vi "Model OPCUA Check Status.vi"(8 "error in (no error)":errorcluster, 11 "Model in":refnum<class "Model.lvclass">) -> (0 "error out":errorcluster)   [LabVIEW 2021, in "Model.lvlib" / "Model.lvclass"]
uses:
  Model.lvclass
  Model.lvclass/Model.ctl
  c082fed2-e689-4666-b91a-ad6a0abfd1cc.vi
  cbdd33bf-e0af-482d-9349-bbda270fe613.vi
  <userlib>/John_Lib/AMC_FW/Read Next Message.vi
  <userlib>/John_Lib/AMC_FW/Parse State Queue__JKI.vi
  <userlib>/John_Lib/AMC_FW/Send Local Message.vi
  <userlib>/John_Lib/AMC_FW/Read Termination Message.vi
  <userlib>/John_Lib/AMC_FW/Create Single Message.vi
  <userlib>/John_Lib/AMC_FW/Update Message Routing Info.vi
  <userlib>/John_Lib/AMC_FW/Globals.vi
  <vilib>/Utility/error.llb/Trim Whitespace.vi
  <userlib>/John_Lib/AMC_FW/String to Array.vi
  <userlib>/John_Lib/AMC_FW/Send Message.vi
  <userlib>/John_Lib/AMC_FW/AMC_FW.lvlib
  <userlib>/John_Lib/OPCUA/OPCUA.lvclass
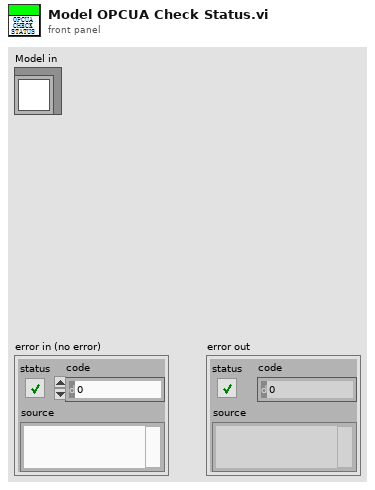
[diagram p1: front panel]
types:
  T1 = typedef "AMC_FW.lvlib/Queue.ctl" = cluster{"Q":T2, "Name":string}
  T2 = typedef "AMC_FW.lvlib/Message Queue.ctl" = refnum<queue>
  T3 = typedef "Model.lvlib/Model.lvclass/DVR.ctl" = cluster{"JKI_Network_Streams":refnum<class "NetworkConnection.lvclass">, "AMC Q":T4}
  T4 = typedef "Model.lvlib/Model.lvclass/AMC Q.ctl" = cluster{"Main":T1, "OPCUA":T1, "NetworkSteam":T1}
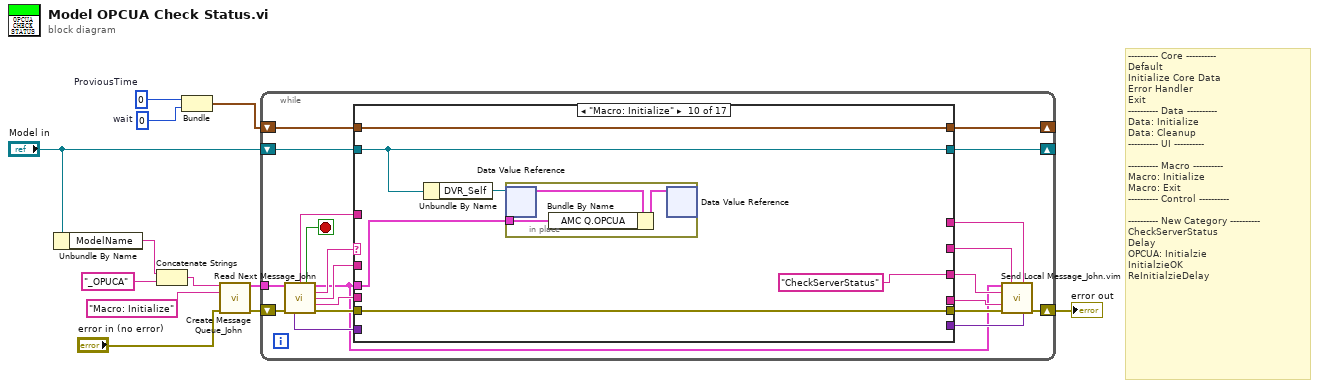
[diagram p0: block diagram]
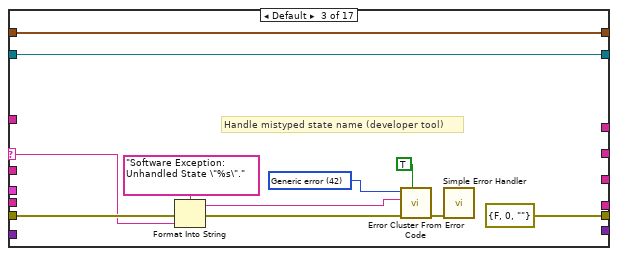
[diagram p4: hidden frame]
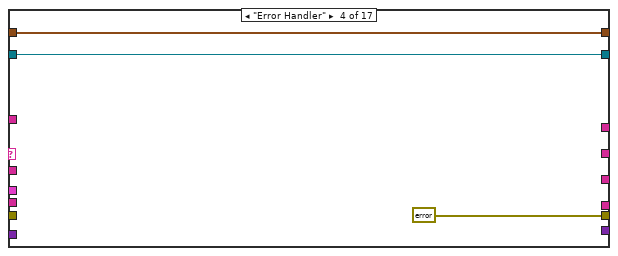
[diagram p5: hidden frame]
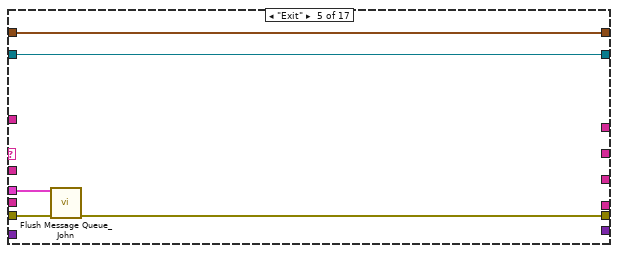
[diagram p6: hidden frame]
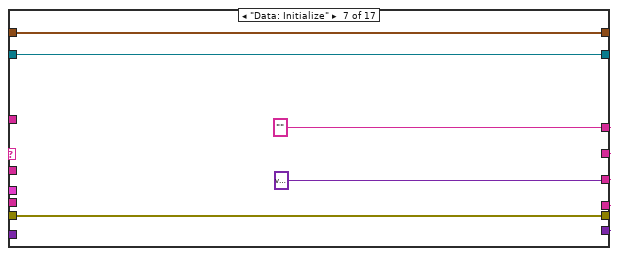
[diagram p8: hidden frame]
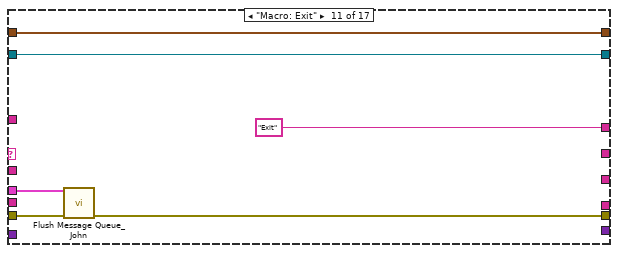
[diagram p11: hidden frame]
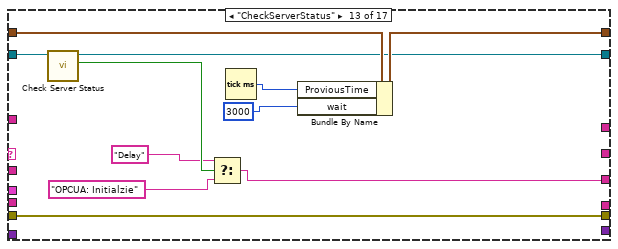
[diagram p13: hidden frame]
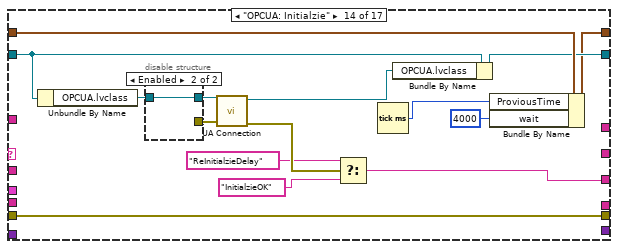
[diagram p14: hidden frame]
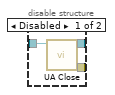
[diagram p15: hidden frame]
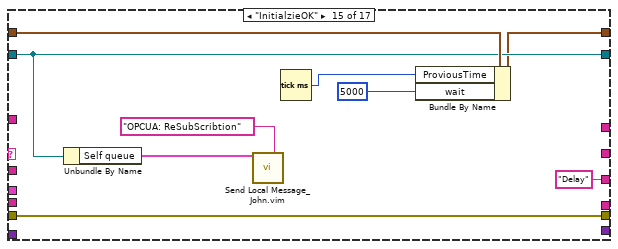
[diagram p16: hidden frame]
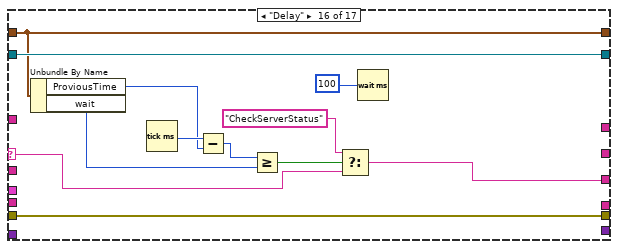
[diagram p17: hidden frame]
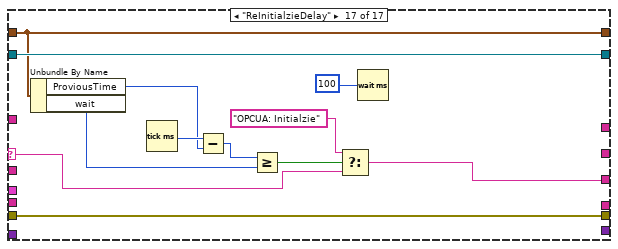
[diagram p18: hidden frame]
diagram:
  w1 = u32 0  # wait
  w11 = u32 0  # ProviousTime
  # "---------- Core ----------\nDefault\nInitialize Core Data\nError Handler\nExit\n---------- Data ----------\nData: Initialize\nData: Cleanup\n---------- UI ----------\n\n---------- Macro ----------\nMacro: Initialize\nMacro: Exit\n---------- Control ----------\n\n---------- New Category ----------\nCheckServerStatus\nDelay\nOPCUA: Initialzie\nInitialzieOK\nReInitialzieDelay"
  n1 = Unbundle By Name("Model in") -> ("ModelName"=w3:string)
  n2 = Concatenate Strings(w3, "_OPUCA" ("string")) -> (w9:string)
  n3 = Bundle("ProviousTime"=w11, "wait"=w1) -> (w10:cluster{"ProviousTime":u32, "wait":u32})  [unwired: 1 in]
  n4 = call <userlib>:"Create Message Queue_John.vi"("message queue name"=w9, "initial message names"="Macro: Initialize", "error in"="error in (no error)") -> ("message queue out"=w7:T1, "error out"=w6:errorcluster)  [unwired: 11 in]
  n5 = while {
    shift-right: [w24] -> w12
    shift-left: w6 -> [w32]
    shift-right: [w33] -> _
    shift-left: "Model in" -> [w26]
    tunnel: w7 -> [w29]
    shift-right: [w14] -> _
    shift-left: w10 -> [w15]
    stop <- w16 stop-if-true
    n6 = call <userlib>:"Read Next Message_John.vi"("Queue In"=w29, "error in"=w32) -> ("Previous State + Arguments"=w25:string, "exit process?"=w16:bool, "Queue Out"=w13:T1, "Current State"=w30:string, "Arguments"=w28:string, "message value"=w27:string, "variant"=w17:variant, "error out"=w31:errorcluster)  [unwired: 4 in, 2 out]
    n7 = case shown="\"Macro: Initialize\"" w30 {
      selector: w30 -> [_ _ w45 _ _ _ _ _ _ _ _ _ _ _ _ w133 w145]
      tunnel: w13 -> [_ _ _ _ w56 _ _ _ _ w73 w87 _ _ _ _ _ _]
      tunnel: w27 -> [_ _ _ _ _ _ _ _ _ _ _ _ _ _ _ _ _]
      tunnel: [w35 w39 errorcluster {"status"=FALSE, "code"=0, "source"=""} ("error out") errorcluster {"status"=FALSE, "code"=0, "source"=""} ("error out") w57 w60 w66 w68 w71 w78 w85 w90 w96 w116 w129 w141 w153] -> w23
      tunnel: w31 -> [w35 w39 w46 _ w58 w60 w66 w68 w71 w78 w86 w90 w96 w116 w129 w141 w153]
      tunnel: w26 -> [w36 w38 w42 w53 w55 w61 w64 w69 w72 w75 w84 w89 w101 w111 w127 w140 w152]
      tunnel: [w36 w38 w42 w53 w55 w61 w64 w69 w72 w75 w84 w89 w97 w110 w127 w140 w152] -> w33
      tunnel: w28 -> [_ _ _ _ _ _ _ _ _ _ _ _ _ _ _ _ _]
      tunnel: w25 -> [_ _ _ _ _ _ _ _ _ _ _ _ _ _ _ _ _]
      tunnel: [_ _ _ _ _ _ w65 _ _ _ _ _ _ _ _ _ _] -> w22
      tunnel: [_ _ _ _ _ _ w65 _ _ _ "Exit" _ _ _ _ _ _] -> w21
      tunnel: [_ _ _ _ _ _ w65 _ _ "CheckServerStatus" _ _ w91 w105 "Delay" ("Previous State + Arguments") w132 w144] -> w20
      tunnel: [_ _ _ _ _ _ w65 _ _ _ _ _ _ _ _ _ _] -> w19
      tunnel: [_ _ _ _ _ _ variant ("variant") _ _ _ _ _ _ _ _ _ _] -> w18
      tunnel: w17 -> [_ _ _ _ _ _ _ _ _ _ _ _ _ _ _ _ _]
      tunnel: w15 -> [w34 w37 w40 w51 w54 w59 w62 w67 w70 w76 w82 w88 w100 w115 w128 w139 w151]
      tunnel: [w34 w37 w40 w51 w54 w59 w62 w67 w70 w76 w82 w88 w99 w104 w123 w139 w151] -> w14
      frame "", "Idle" {
      }
      frame "---------- Core ----------" {
      }
      frame Default {
        w48 = 42 items=["No error", "Argument error", "Memory is full", "Out of zone", "End of file", "File already open", "Generic file I/O error", "File not found", "File permission error", "Disk is full", "Duplicate path", "Too many files open", "System feature not enabled", "Resource file not found", "Cannot add resource", "Resource not found", "Image not found", "Image memory error", "Pen does not exist", "Config type invalid", "Config token not found", "Config parse error", "Config memory error", "Bad external code format", "Bad external code offset", "External code not present", "Null window", "Destroy window error", "Null menu", "Print aborted", "Bad print record", "Print driver error", "Windows error during printing", "Memory error during printing", "Print dialog error", "Generic print error", "Invalid device refnum", "Device not found", "Device parameter error", "Device unit error", "Cannot open device", "Device call aborted", "Generic error", "Cancelled by user", "Object ID too low", "Object ID too high", "Object not in heap", "Unknown heap", "Unknown object (invalid DefProc)", "Unknown object (DefProc not in table)", "Message out of range", "Invalid (null) method", "Unknown message", "Manager call not supported", "Bad address", "Network operation in progress", "Network operation timed out", "Connection is busy", "Network attribute not supported", "Network error", "Address in use", "System out of memory", "Connection aborted", "Connection refused", "Not connected", "Already connected", "Connection closed", "Initialization error (interapplication manager)", "Bad occurrence", "Wait on unbound occurrence handler", "Occurrence queue overflow", "Datalog type conflict", "Unused", "Unrecognized type (interapplication manager)", "Memory corrupt", "Failed to make temporary DLL", "Old CIN version", "Drag socket not found", "Failed to load drop-object", "Failed to register OLE object", "Failed to release OLE object", "Format specifier type mismatch", "Unknown format specifier", "Too few format specifiers", "Too many format specifiers", "Scan failed", "Newer CIN version", "Error converting to variant", "Runtime menu error", "Password tampered", "Variant attribute not found", "Incompatible variant data type", "Event data is not available", "Event Store is not present", "Occurrence is not found", "Event Queue is not created", "Event info is not available", "Refnum passed is NULL", "Error retrieving Class GUID", "Error retrieving CoClass GUID", "Error retrieving TypeLib GUID.", "Bad built application magic bytes.", "Specific driver is different from the specific driver associated with the Logical Name.", "There is no session opened to the class driver.", "Max Error", "MAX - Error with config objects", "MAX - Error loading configuration", "MAX - Group not supported"]
        # "Handle mistyped state name (developer tool)"
        n8 = Format Into String(format string="Software Exception: Unhandled State \"%s\"." ("message"), error in=w46, w45) -> (resulting string=w41:string, error out=w49:errorcluster)  [unwired: 1 in]
        n9 = call <vilib>:"Error Cluster From Error Code.vi"("show call chain? (False)"=TRUE, "error in (no error)"=w49, "error message (\"\")"=w41, "error code (0)"=w48) -> ("error out"=w44:errorcluster)  [unwired: 5 in]
        n10 = call <vilib>:"Simple Error Handler.vi"("error in (no error)"=w44) -> ()  [unwired: 4 in, 5 out]
      }
      frame "Error Handler" {
      }
      frame "Exit" {
        n11 = call <userlib>:"Flush Message Queue_John.vi"("Queue In"=w56, "error in"=w58) -> ("error out"=w57:errorcluster)  [unwired: 11 in, 2 out]
      }
      frame "---------- Data ----------" {
      }
      frame "Data: Initialize" {
        w65 = "" ("Elements in Front")
      }
      frame "---------- UI ----------" {
      }
      frame "---------- Macro ----------" {
      }
      frame "Macro: Initialize" {
        n12 = Unbundle By Name(w75) -> ("DVR_Self"=w74:refnum<data-value>)
        n13 = in-place {
          in-place-border: w73 -> [w79]
          n14 = in-place-dvr #1(w74) -> (w81:T3)  [unwired: 1 out]
          n15 = Bundle By Name(cluster=w81, "AMC Q.OPCUA"=w79) -> (w80:T3)
          n16 = in-place-dvr #1(w80) -> ()  [unwired: 2 out]
        }
      }
      frame "Macro: Exit" {
        n17 = call <userlib>:"Flush Message Queue_John.vi"("Queue In"=w87, "error in"=w86) -> ("error out"=w85:errorcluster)  [unwired: 11 in, 2 out]
      }
      frame "---------- Control ----------" {
      }
      frame "CheckServerStatus" {
        n18 = call "Check Server Status.vi"("Model in"=w101) -> ("T: OK"=w95:bool, "Model out"=w97:refnum<class "Model.lvclass">)  [unwired: 8 in, 1 out]
        n19 = Select(t="Delay" ("Elements in Front"), s=w95, f="OPCUA: Initialzie" ("Elements in Front")) -> (s? t:f=w91:string)
        n20 = Tick Count (ms)() -> (millisecond timer value=w98:u32)
        n21 = Bundle By Name(cluster=w100, "ProviousTime"=w98, "wait"=u32 3000 ("t")) -> (w99:cluster{"ProviousTime":u32, "wait":u32})
      }
      frame "OPCUA: Initialzie" {
        n22 = Unbundle By Name(w111) -> ("OPCUA.lvclass"=w113:refnum<class "OPCUA.lvclass">)
        n23 = disable-structure shown="Enabled" {
          disable-tunnel: [w119 _] -> w114
          disable-tunnel: w113 -> [w118 w120]
          disable-tunnel: [w117 w120] -> w112
          frame Disabled {
            n24 = call <userlib>:"UA Close.vi"("OPCUA in"=w118) -> ("error out"=w119:errorcluster, "OPCUA out"=w117:refnum<class "OPCUA.lvclass">)  [unwired: 9 in]
          }
          frame Enabled {
          }
        }
        n25 = call <userlib>:"UA Connection.vi"("error in (no error)"=w114, "OPCUA in"=w112) -> ("error out"=w108:errorcluster, "OPCUA out"=w109:refnum<class "OPCUA.lvclass">)  [unwired: 8 in]
        n26 = Select(t="ReInitialzieDelay" ("string"), s=w108, f="InitialzieOK") -> (s? t:f=w105:string)
        n27 = Tick Count (ms)() -> (millisecond timer value=w103:u32)
        n28 = Bundle By Name(cluster=w111, "OPCUA.lvclass"=w109) -> (w110:refnum<class "Model.lvclass">)
        n29 = Bundle By Name(cluster=w115, "ProviousTime"=w103, "wait"=u32 4000) -> (w104:cluster{"ProviousTime":u32, "wait":u32})
      }
      frame "InitialzieOK" {
        n30 = Unbundle By Name(w127) -> ("Self queue"=w126:T1)
        n31 = call "Send Local Message_John.vim"("Queue In"=w126, "Elements in Front"="OPCUA: ReSubScribtion") -> ()  [unwired: 11 in, 3 out]
        n32 = Tick Count (ms)() -> (millisecond timer value=w121:u32)
        n33 = Bundle By Name(cluster=w128, "ProviousTime"=w121, "wait"=u32 5000) -> (w123:cluster{"ProviousTime":u32, "wait":u32})
      }
      frame "Delay" {
        n34 = Unbundle By Name(w139) -> ("ProviousTime"=w137:u32, "wait"=w130:u32)
        n35 = Tick Count (ms)() -> (millisecond timer value=w138:u32)
        n36 = Subtract(x=w138, y=w137) -> (x-y=w136:u32)
        n37 = Greater Or Equal?(x=w136, y=w130) -> (x >= y?=w135:bool)
        n38 = Select(t="CheckServerStatus" ("Previous State + Arguments"), s=w135, f=w133) -> (s? t:f=w132:string)
        n39 = Wait (ms)(milliseconds to wait=u32 100) -> ()  [unwired: 1 out]
      }
      frame "ReInitialzieDelay" {
        n40 = Unbundle By Name(w151) -> ("ProviousTime"=w149:u32, "wait"=w142:u32)
        n41 = Tick Count (ms)() -> (millisecond timer value=w150:u32)
        n42 = Subtract(x=w150, y=w149) -> (x-y=w148:u32)
        n43 = Greater Or Equal?(x=w148, y=w142) -> (x >= y?=w147:bool)
        n44 = Select(t="OPCUA: Initialzie" ("Previous State + Arguments"), s=w147, f=w145) -> (s? t:f=w144:string)
        n45 = Wait (ms)(milliseconds to wait=u32 100) -> ()  [unwired: 1 out]
      }
    }
    n46 = call "Send Local Message_John.vim"("Queue In"=w13, "receiver process (\"\" - local)"=w22, "Elements in Front"=w21, "Elements at Back"=w20, "message value"=w19, "error in"=w23, "variant"=w18) -> ("error out"=w24:errorcluster)  [unwired: 6 in, 2 out]
  }
  "error out" <- w12
